vi "6.vi"() -> ()   [LabVIEW 2017]
panel:
  out "Waveform Chart":u32(graph)
  in  "stop":bool
  out "Gauge":dbl(knob) scale=0.0..255.0
  out "Thermometer":dbl(slide) scale=0.0..255.0
  out "Numeric":dbl
  in  "Array":bool[](array[boolean])
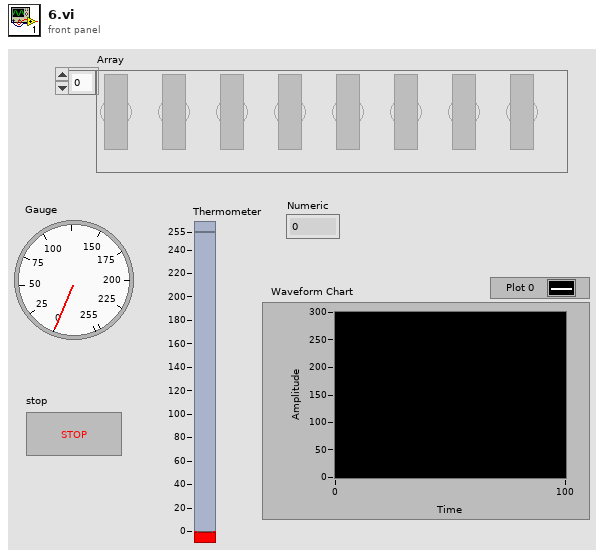
[diagram p1: front panel]
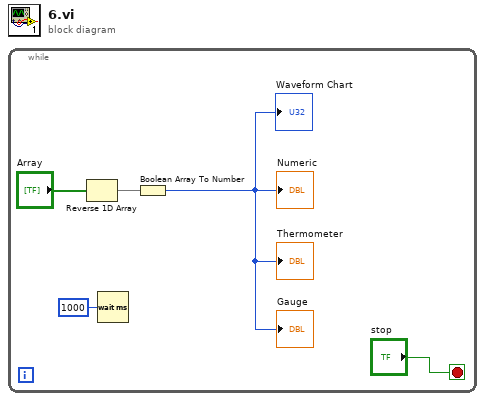
[diagram p0: block diagram]
diagram:
  n1 = while {
    stop <- "stop" stop-if-true
    n2 = Reverse 1D Array(array="Array") -> (reversed array=w3:bool[])
    n3 = Wait (ms)(milliseconds to wait=u32 1000) -> ()  [unwired: 1 out]
    n4 = Boolean Array To Number(Boolean array=w3) -> (number=→"Numeric" →"Thermometer" →"Gauge" →"Waveform Chart":u32)
  }
